vi "Update BBM Chuck Status.vi"(10 "BM Chuck Control":T1={"Slot 1"={"Populated?"=TRUE}, "Slot 2"={"Populated?"=TRUE}, "Slot 3"={"Populated?"=TRUE}, "Slot 4"={"Populated?"=TRUE}}, 11 "BBM chuck reference":refnum<vi>) -> ()   [LabVIEW 2011]
uses:
  UI typedefs/BM Chuck Control.ctl
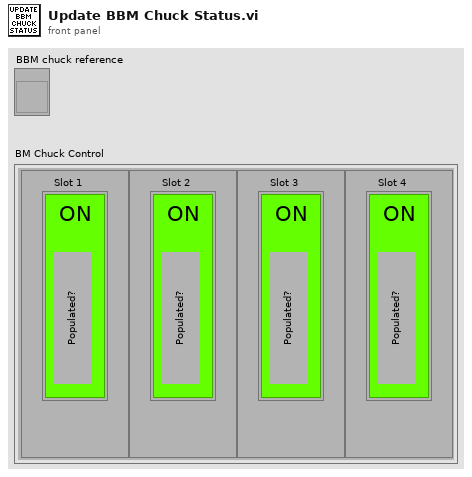
[diagram p1: front panel]
types:
  T1 = typedef "BM Chuck Control.ctl" = cluster{"Slot 1":cluster{"Populated?":bool}, "Slot 2":cluster{"Populated?":bool}, "Slot 3":cluster{"Populated?":bool}, "Slot 4":cluster{"Populated?":bool}}
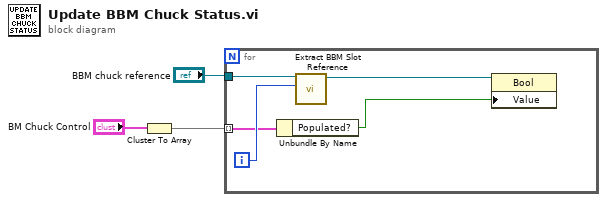
[diagram p0: block diagram]
diagram:
  n1 = Cluster To Array(cluster="BM Chuck Control") -> (array=w1:cluster{"Populated?":bool}[])
  n2 = for {
    tunnel: "BBM chuck reference" -> [w8]
    tunnel: w1 -> [w6] mode=indexing
    i -> [w7]
    n3 = Unbundle By Name(w6) -> ("Populated?"=w4:bool)
    n4 = call "Extract BBM Slot Reference.vi"("Slot"=w7, "Cluster in"=w8) -> ("Populated Reference"=w5:refnum<vi>)  [unwired: 9 in]
    n5 = property class="Bool"(reference=w5, "Value"=w4) -> ()  [unwired: 1 in, 2 out]
  }
